vi "Error Message.vi"() -> ()   [LabVIEW 2017, in "Assertions.Tests.lvlib" / "Assert String Contains String Ignoring Case.lvlib"]
uses:
  Assert String Contains String Ignoring Case.lvlib
  src/Transparent Assertions/Assertions/Assertions.lvlib
panel:
  out "error out":errorcluster
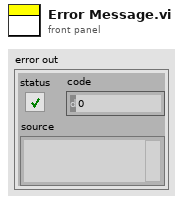
[diagram p1: front panel]
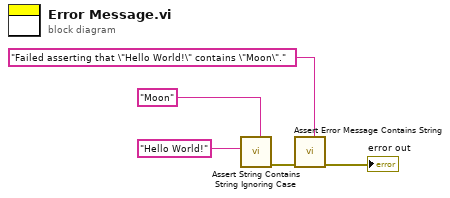
[diagram p0: block diagram]
diagram:
  n1 = call "Assert String Contains String Ignoring Case.vi"("Needle"="Moon", "Haystack"="Hello World!") -> ("error out"=w1:errorcluster)  [unwired: 9 in]
  n2 = call "Assert Error Message Contains String.vi"("Expected"="Failed asserting that \"Hello World!\" contains \"Moon\".", "error in (no error)"=w1) -> ("error out"=→"error out":errorcluster)  [unwired: 9 in]
